vi "TEST - Get Cluster Element by Name.vi"(8 "error in (no error)":errorcluster) -> (0 "error out":errorcluster, 2 "pass":bool)   [LabVIEW 2020]
uses:
  source/library/oglib_lvdata.lvlib
panel:
  out "Failures":T1(array[cluster])
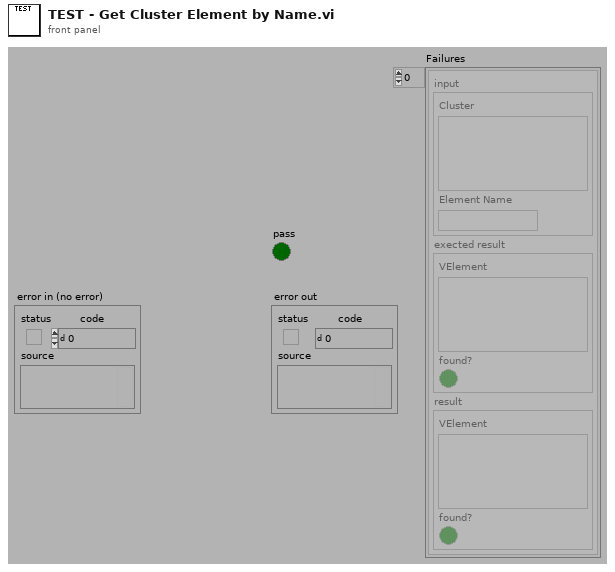
[diagram p1: front panel]
types:
  T1 = cluster{"input":cluster{"Cluster":variant, "Element Name":string}, "exected result":cluster{"VElement":variant, "found?":bool}, "result":cluster{"VElement":variant, "found?":bool}}[]
  T2 = cluster{"input":cluster{"Cluster":variant, "Element Name":string}, "exected result":cluster{"VElement":variant, "found?":bool}, "result":cluster{"VElement":variant, "found?":bool}}
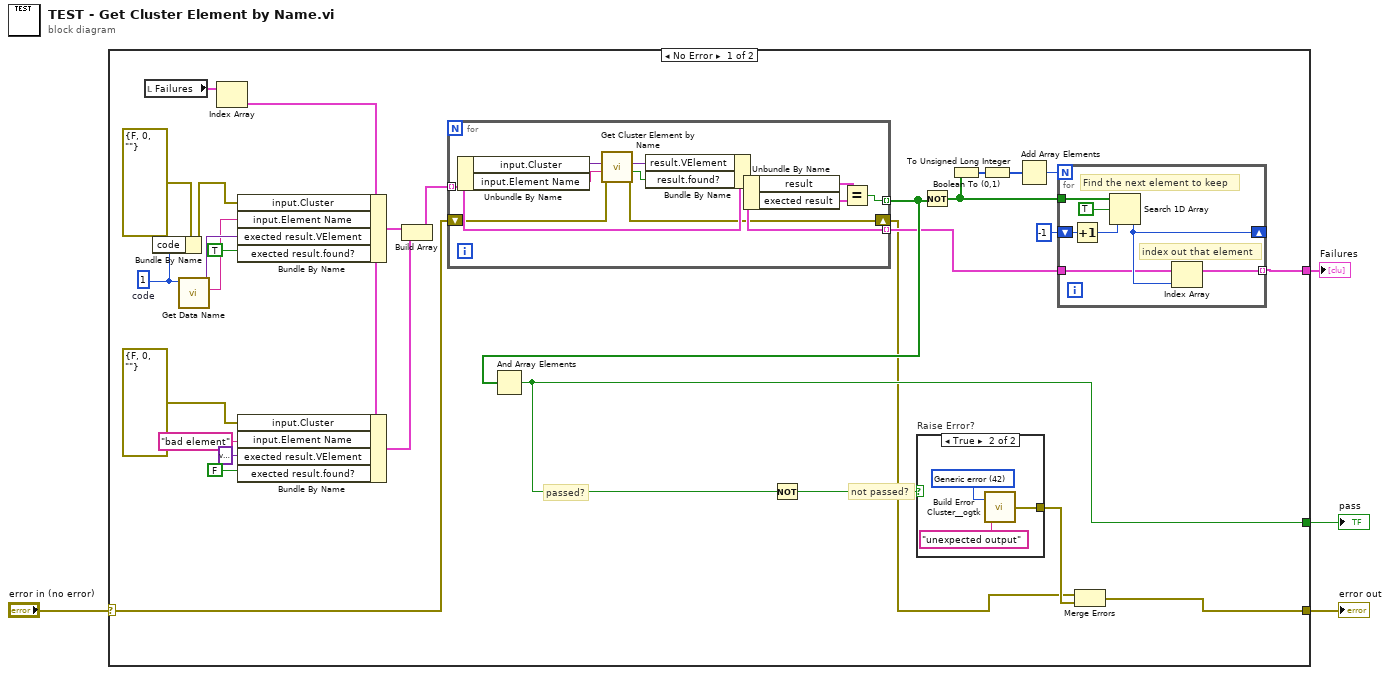
[diagram p0: block diagram]
diagram:
  n1 = case shown="No Error" "error in (no error)" {
    selector: "error in (no error)" -> [w19 w55]
    tunnel: [w30 _] -> w4
    tunnel: [w33 w55] -> w2
    tunnel: [w22 _] -> w1
    frame No Error {
      w11 = 1  # code
      # "not passed?"
      # "passed?"
      n2 = local read "Failures"() -> (w17:T1)
      n3 = Bundle By Name(cluster=errorcluster {"status"=FALSE, "code"=0, "source"=""} ("error in (no error)"), "code"=w11) -> (w12:errorcluster)
      n4 = call "Get Data Name.vi"("Data"=w11) -> ("Data Name"=w15:string, "Data dup"=w16:variant)  [unwired: 8 in, 1 out]
      n5 = Index Array(array=w17) -> (element=w8:T2)  [unwired: 1 in]
      n6 = Bundle By Name(cluster=w8, "input.Cluster"=w12, "input.Element Name"=w15, "exected result.VElement"=w16, "exected result.found?"=TRUE) -> (w21:T2)
      n7 = Bundle By Name(cluster=w8, "input.Cluster"=errorcluster {"status"=FALSE, "code"=0, "source"=""} ("error in (no error)"), "input.Element Name"="bad element", "exected result.VElement"=variant, "exected result.found?"=FALSE) -> (w7:T2)
      n8 = Build Array(w21, w7) -> (w20:T1)
      n9 = for {
        tunnel: w20 -> [w50] mode=indexing
        tunnel: [w51] -> w24 mode=indexing
        tunnel: [w49] -> w23 mode=indexing
        shift-right: [w44] -> w18
        shift-left: w19 -> [w45]
        n10 = Unbundle By Name(w50) -> ("input.Cluster"=w46:variant, "input.Element Name"=w43:string)
        n11 = call "Get Cluster Element by Name.vi"("error in (no error)"=w45, "Element Name"=w43, "Cluster"=w46) -> ("error out"=w44:errorcluster, "found?"=w41:bool, "VElement"=w42:variant)  [unwired: 6 in]
        n12 = Bundle By Name(cluster=w50, "result.VElement"=w42, "result.found?"=w41) -> (w49:T2)
        n13 = Unbundle By Name(w49) -> ("result"=w48:cluster{"VElement":variant, "found?":bool}, "exected result"=w47:cluster{"VElement":variant, "found?":bool})
        n14 = Equal?(x=w48, y=w47) -> (x = y?=w51:bool)
      }
      n15 = And Array Elements(Boolean array=w24) -> (logical AND=w30:bool)
      n16 = Not(x=w30) -> (.not. x?=w31:bool)
      n17 = case "Raise Error?" shown="True" w31 {
        tunnel: [_ w52] -> w32
        frame False {
        }
        frame True {
          w53 = 42 items=["No error", "Argument error", "Memory is full", "Out of zone", "End of file", "File already open", "Generic file I/O error", "File not found", "File permission error", "Disk is full", "Duplicate path", "Too many files open", "System feature not enabled", "Resource file not found", "Cannot add resource", "Resource not found", "Image not found", "Image memory error", "Pen does not exist", "Config type invalid", "Config token not found", "Config parse error", "Config memory error", "Bad external code format", "Bad external code offset", "External code not present", "Null window", "Destroy window error", "Null menu", "Print aborted", "Bad print record", "Print driver error", "Windows error during printing", "Memory error during printing", "Print dialog error", "Generic print error", "Invalid device refnum", "Device not found", "Device parameter error", "Device unit error", "Cannot open device", "Device call aborted", "Generic error", "Cancelled by user", "Object ID too low", "Object ID too high", "Object not in heap", "Unknown heap", "Unknown object (invalid DefProc)", "Unknown object (DefProc not in table)", "Message out of range", "Invalid (null) method", "Unknown message", "Manager call not supported", "Bad address", "Network operation in progress", "Network operation timed out", "Connection is busy", "Network attribute not supported", "Network error", "Address in use", "System out of memory", "Connection aborted", "Connection refused", "Not connected", "Already connected", "Connection closed", "Initialization error (interapplication manager)", "Bad occurrence", "Wait on unbound occurrence handler", "Occurrence queue overflow", "Datalog type conflict", "Unused", "Unrecognized type (interapplication manager)", "Memory corrupt", "Failed to make temporary DLL", "Old CIN version", "Drag socket not found", "Failed to load drop-object", "Failed to register OLE object", "Failed to release OLE object", "Format specifier type mismatch", "Unknown format specifier", "Too few format specifiers", "Too many format specifiers", "Scan failed", "Newer CIN version", "Error converting to variant", "Runtime menu error", "Password tampered", "Variant attribute not found", "Incompatible variant data type", "Event data is not available", "Event Store is not present", "Occurrence is not found", "Event Queue is not created", "Event info is not available", "Refnum passed is NULL", "Error retrieving Class GUID", "Error retrieving CoClass GUID", "Error retrieving TypeLib GUID.", "Bad built application magic bytes.", "Specific driver is different from the specific driver associated with the Logical Name.", "There is no session opened to the class driver.", "Max Error", "MAX - Error with config objects", "MAX - Error loading configuration", "MAX - Group not supported"]
          n18 = call <userlib>:"Build Error Cluster__ogtk.vi"("String to Prepend to source (\"\")"="unexpected output" ("String to Prepend to source (\"\")"), "code"=w53) -> ("error out"=w52:errorcluster)
        }
      }
      n19 = Not(x=w24) -> (.not. x?=w26:bool[])
      n20 = Boolean To (0,1)(Boolean=w26) -> (0, 1=w27:i16[])
      n21 = To Unsigned Long Integer(number=w27) -> (unsigned 32bit integer=w25:u32[])
      n22 = Add Array Elements(numeric array=w25) -> (sum=w28:u32)
      n23 = for {
        N: w28 -> [_]
        tunnel: w23 -> [w36]
        tunnel: w26 -> [w40]
        shift-right: [w37] -> _
        shift-left: -1 ("start index (0)") -> [w38]
        tunnel: [w35] -> w22 mode=indexing
        # "index out that element"
        # "Find the next element to keep"
        n24 = Increment(x=w38) -> (x+1=w34:i32)
        n25 = Search 1D Array(1D array=w40, element=TRUE, start index (0)=w34) -> (index of element=w37:i32)
        n26 = Index Array(array=w36, index=w37) -> (element=w35:T2)
      }
      n27 = Merge Errors(w18, w32) -> (w33:errorcluster)
    }
    frame Error {
    }
  }
  "pass" <- w4
  "error out" <- w2
  "Failures" <- w1
